vi "Validate Reference by GUID.vi"(8 "error in":errorcluster, 9 "name":string, 10 "valid guids":string[](array[string]), 11 "item in":T1 format="%.0x") -> (0 "error out":errorcluster, 3 "item out":T1 format="%.0x")   [LabVIEW 2020, in "Routing and Faulting Scripting.lvlib"]
uses:
  Routing and Faulting Scripting.lvlib
  <vilib>/NI VeriStand/Custom Device API/Custom Device Item Ref.ctl
  NationalInstruments.VeriStand.SystemDefinitionAPI
  <vilib>/NI VeriStand/Custom Device API/Custom Device API.lvlib
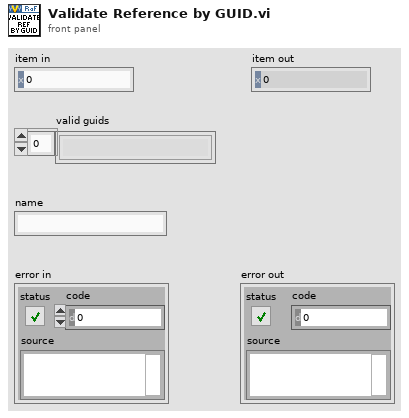
[diagram p1: front panel]
types:
  T1 = typedef "Custom Device API.lvlib/Custom Device Item Ref.ctl" = u64
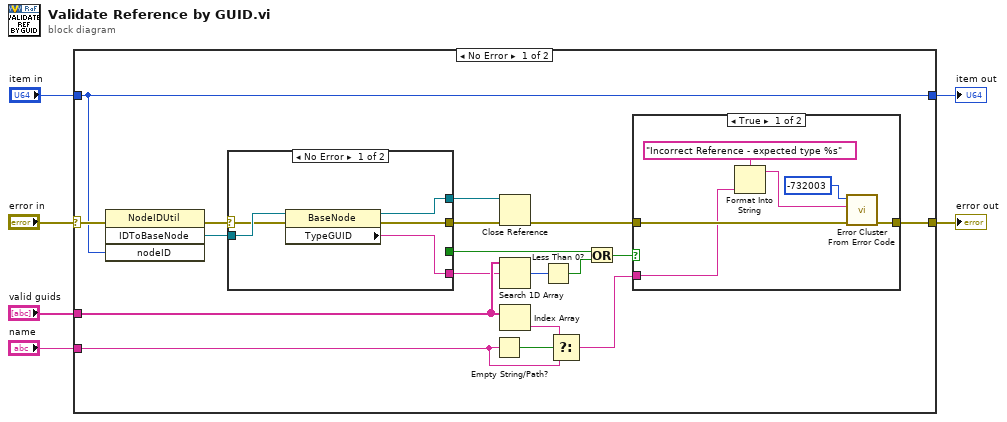
[diagram p0: block diagram]
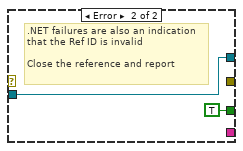
[diagram p2: hidden frame]
diagram:
  n1 = case shown="No Error" "error in" {
    selector: "error in" -> [w16 w40]
    tunnel: [w24 w40] -> w6
    tunnel: "item in" -> [w11 w39]
    tunnel: "name" -> [w22 _]
    tunnel: "valid guids" -> [w20 _]
    tunnel: [w11 w39] -> w3
    frame No Error {
      n2 = invoke class="NodeIDUtil" method="IDToBaseNode"(error in=w16, "nodeID"=w11) -> (error out=w17:errorcluster, "IDToBaseNode"=w18:refnum<k24>)  [unwired: 2 in, 2 out]
      n3 = case shown="No Error" w17 {
        selector: w17 -> [w25 _]
        tunnel: [w29 _] -> w14
        tunnel: [w28 _] -> w15
        tunnel: [w27 w31] -> w12
        tunnel: w18 -> [w26 w31]
        tunnel: [_ TRUE] -> w8
        frame No Error {
          n4 = property class="BaseNode"(reference=w26, error in=w25) -> (reference out=w27:refnum<k24>, error out=w28:errorcluster, "TypeGUID"=w29:string)
        }
        frame Error {
          # ".NET failures are also an indication\nthat the Ref ID is invalid\n\nClose the reference and report"
        }
      }
      n5 = Empty String/Path?(string/path=w22) -> (empty?=w23:bool)
      n6 = Close Reference(reference=w12, error in (no error)=w15) -> (error out=w13:errorcluster)
      n7 = Search 1D Array(1D array=w20, element=w14) -> (index of element=w10:i32)  [unwired: 1 in]
      n8 = Index Array(array=w20) -> (element=w19:string)  [unwired: 1 in]
      n9 = Less Than 0?(x=w10) -> (x < 0?=w9:bool)
      n10 = Select(t=w19, s=w23, f=w22) -> (s? t:f=w21:string)
      n11 = Or(x=w8, y=w9) -> (x .or. y?=w7:bool)
      n12 = case shown="True" w7 {
        tunnel: w13 -> [w36 w38]
        tunnel: [w35 w38] -> w24
        tunnel: w21 -> [w33 _]
        frame True {
          n13 = Format Into String(format string="Incorrect Reference - expected type %s" ("error message (\"\")"), w33) -> (resulting string=w32:string)  [unwired: 2 in, 1 out]
          n14 = call <vilib>:"Error Cluster From Error Code.vi"("error in (no error)"=w36, "error message (\"\")"=w32, "error code (0)"=-732003) -> ("error out"=w35:errorcluster)  [unwired: 6 in]
        }
        frame False {
        }
      }
    }
    frame Error {
    }
  }
  "error out" <- w6
  "item out" <- w3
